vi "Example 01.vi"   [LabVIEW 2016]
uses:
  Hardware/Parent/Hardware.lvclass
  Hardware/DAQmx/DAQmx.lvclass
  Hardware/Simulated/Simulated.lvclass
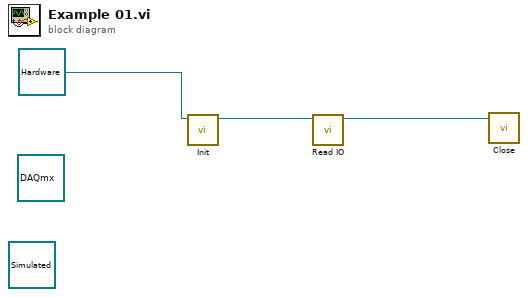
[diagram p0: block diagram]
diagram:
  (unwired) refnum<class "Simulated.lvclass"> refnum ("Simulated.lvclass")
  (unwired) refnum<class "DAQmx.lvclass"> refnum ("DAQmx.lvclass")
  n1 = call-dynamic "Init.vi"("Hardware in"=refnum<class "Hardware.lvclass"> refnum ("Hardware.lvclass")) -> ("Hardware out"=w3:refnum<class "Hardware.lvclass">)  [unwired: 9 in, 1 out]
  n2 = call-dynamic "Read IO.vi"("Hardware in"=w3) -> ("Hardware out"=w2:refnum<class "Hardware.lvclass">)  [unwired: 9 in, 1 out]
  n3 = call-dynamic "Close.vi"("Hardware in"=w2) -> ()  [unwired: 9 in, 2 out]
